vi "set Position.vi"(10 "Position":refnum<class "Vector 2D.lvclass">, 11 "Motion in":refnum<class "Motion.lvclass">) -> (3 "Motion out":refnum<class "Motion.lvclass">)   [LabVIEW 2021, in "Motion.lvclass"]
uses:
  Motion.lvclass
  Re-use Libraries/Vector 2D/Vector 2D.lvclass
  Motion.lvclass/Motion.ctl
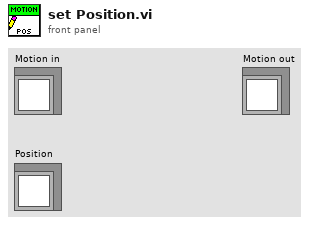
[diagram p1: front panel]
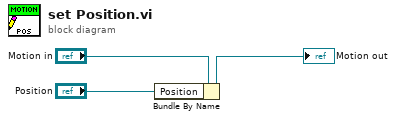
[diagram p0: block diagram]
diagram:
  n1 = Bundle By Name(cluster="Motion in", "Position"="Position") -> (→"Motion out":refnum<class "Motion.lvclass">)
